vi "Write Item Indent.vi"(10 "Item Indent":i32, 11 "BetterTreeItem in":refnum<class "BetterItem.lvclass">) -> (3 "BetterTreeItem out":refnum<class "BetterItem.lvclass">)   [LabVIEW 2020, in "BetterDragAndDrop.lvlib" / "BetterItem.lvclass"]
uses:
  BetterItem.lvclass
  BetterItem.lvclass/BetterItem.ctl
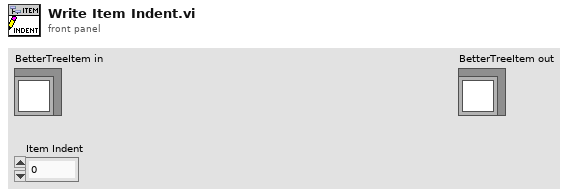
[diagram p1: front panel]
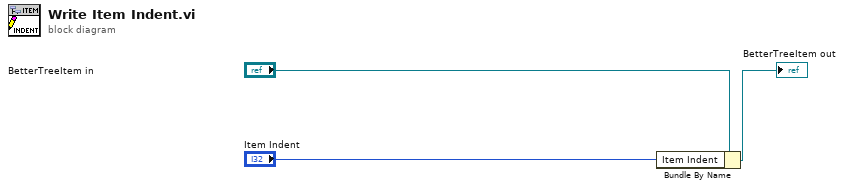
[diagram p0: block diagram]
diagram:
  n1 = Bundle By Name(cluster="BetterTreeItem in", "Item Indent"="Item Indent") -> (→"BetterTreeItem out":refnum<class "BetterItem.lvclass">)
